vi "Outputs.vi"(8 "error in (no error)":errorcluster, 11 "State in":T1={"State"=enum."Idle", "Start Time"=timestamp(0 s since 1904-01-01), "Configuration"={"Cycle Period"=0.0, "PID 2 Parameters"={"Input Device"=enum."4-20mA", "Output Device"=enum."Default", "Setpoint"=0.0, "PID gains"={"proportional gain (Kc)"=0.0, "integral time (Ti, min)"=0.0, "derivative time (Td, min)"=100.0}, "output range"={"output low"=0.0, "output high"=1.0}}, "Manual Entry"=0.0, "Auto?"=TRUE, "4-20mA Input Settings"={"Input Channel "=0}, "4-20mA Out Settings"={"Output DAQ Task"=""}, "Input Channel Tag Name "=""}, "Current Time"=timestamp(0 s since 1904-01-01), "PID 1 Parameters"={"Setpoint"=0.0, "PID gains"={"proportional gain (Kc)"=1.0, "integral time (Ti, min)"=0.01, "derivative time (Td, min)"=0.0}}, "First Iteration"=FALSE, "Data"={"4-20mA Input"=0.0, "PID 2 Process Variable"=0.0, "PID 2 Output"=0.0, "4-20mA Output"=0.0}, "Process Name"="", "Pump On?"=enum."Off", "Input Error"=FALSE, "Output Error"=FALSE, "Log Started"=FALSE, "Current Setpoint"=0.0} {"Configuration"."PID 2 Parameters"."output range"."output low" format="%.2f"; "Configuration"."PID 2 Parameters"."output range"."output high" min=0.0 max=100.0 format="%.2f"; "Configuration"."PID 2 Parameters"."PID gains"."derivative time (Td, min)" format="%.3f"; "Configuration"."PID 2 Parameters"."PID gains"."integral time (Ti, min)" format="%.3f"; "Configuration"."PID 2 Parameters"."PID gains"."proportional gain (Kc)" format="%.3f"; "PID 1 Parameters"."PID gains"."derivative time (Td, min)" format="%.3f"; "PID 1 Parameters"."PID gains"."integral time (Ti, min)" format="%.3f"; "PID 1 Parameters"."PID gains"."proportional gain (Kc)" format="%.3f"}) -> (0 "error out":errorcluster, 3 "State out":T1={"State"=enum."Idle", "Start Time"=timestamp(0 s since 1904-01-01), "Configuration"={"Cycle Period"=0.0, "PID 2 Parameters"={"Input Device"=enum."4-20mA", "Output Device"=enum."Default", "Setpoint"=0.0, "PID gains"={"proportional gain (Kc)"=0.0, "integral time (Ti, min)"=0.0, "derivative time (Td, min)"=100.0}, "output range"={"output low"=0.0, "output high"=1.0}}, "Manual Entry"=0.0, "Auto?"=TRUE, "4-20mA Input Settings"={"Input Channel "=0}, "4-20mA Out Settings"={"Output DAQ Task"=""}, "Input Channel Tag Name "=""}, "Current Time"=timestamp(0 s since 1904-01-01), "PID 1 Parameters"={"Setpoint"=0.0, "PID gains"={"proportional gain (Kc)"=1.0, "integral time (Ti, min)"=0.01, "derivative time (Td, min)"=0.0}}, "First Iteration"=FALSE, "Data"={"4-20mA Input"=0.0, "PID 2 Process Variable"=0.0, "PID 2 Output"=0.0, "4-20mA Output"=0.0}, "Process Name"="", "Pump On?"=enum."Off", "Input Error"=FALSE, "Output Error"=FALSE, "Log Started"=FALSE, "Current Setpoint"=0.0} {"Configuration"."PID 2 Parameters"."output range"."output low" format="%.2f"; "Configuration"."PID 2 Parameters"."output range"."output high" min=0.0 max=100.0 format="%.2f"; "Configuration"."PID 2 Parameters"."PID gains"."derivative time (Td, min)" format="%.3f"; "Configuration"."PID 2 Parameters"."PID gains"."integral time (Ti, min)" format="%.3f"; "Configuration"."PID 2 Parameters"."PID gains"."proportional gain (Kc)" format="%.3f"; "PID 1 Parameters"."PID gains"."derivative time (Td, min)" format="%.3f"; "PID 1 Parameters"."PID gains"."integral time (Ti, min)" format="%.3f"; "PID 1 Parameters"."PID gains"."proportional gain (Kc)" format="%.3f"})   [LabVIEW 2018, in "4-20mA Module.lvlib" / "4-20mA Module Engine.lvlib"]
uses:
  4-20mA Module Engine.lvlib
  State Cluster.ctl
  State Enum.ctl
  Pressure Transmitter/Pressure Transmitter Device Settings.ctl
  Pressure Reg Module/Pressure Regulator Device Settings.ctl
  Measure Instrument/PID 1 Parameters Cluster.ctl
  Tag VIs/Tag FGV Operation Enum.ctl
  Shared Variables/Dynamic Shared Variables.lvlib
  Pressure Reg Module/Pressure Regulator Library.lvlib
  Flow Regulator/Pressure Reg Module/Flow Regulator Library.lvlib
  Pressure Transmitter/Pressure Transmitter Library.lvlib
panel:
  # "Instrument Settings"
  # "Instrument Settings"
  # "Instrument Settings"
  # "Instrument Settings"
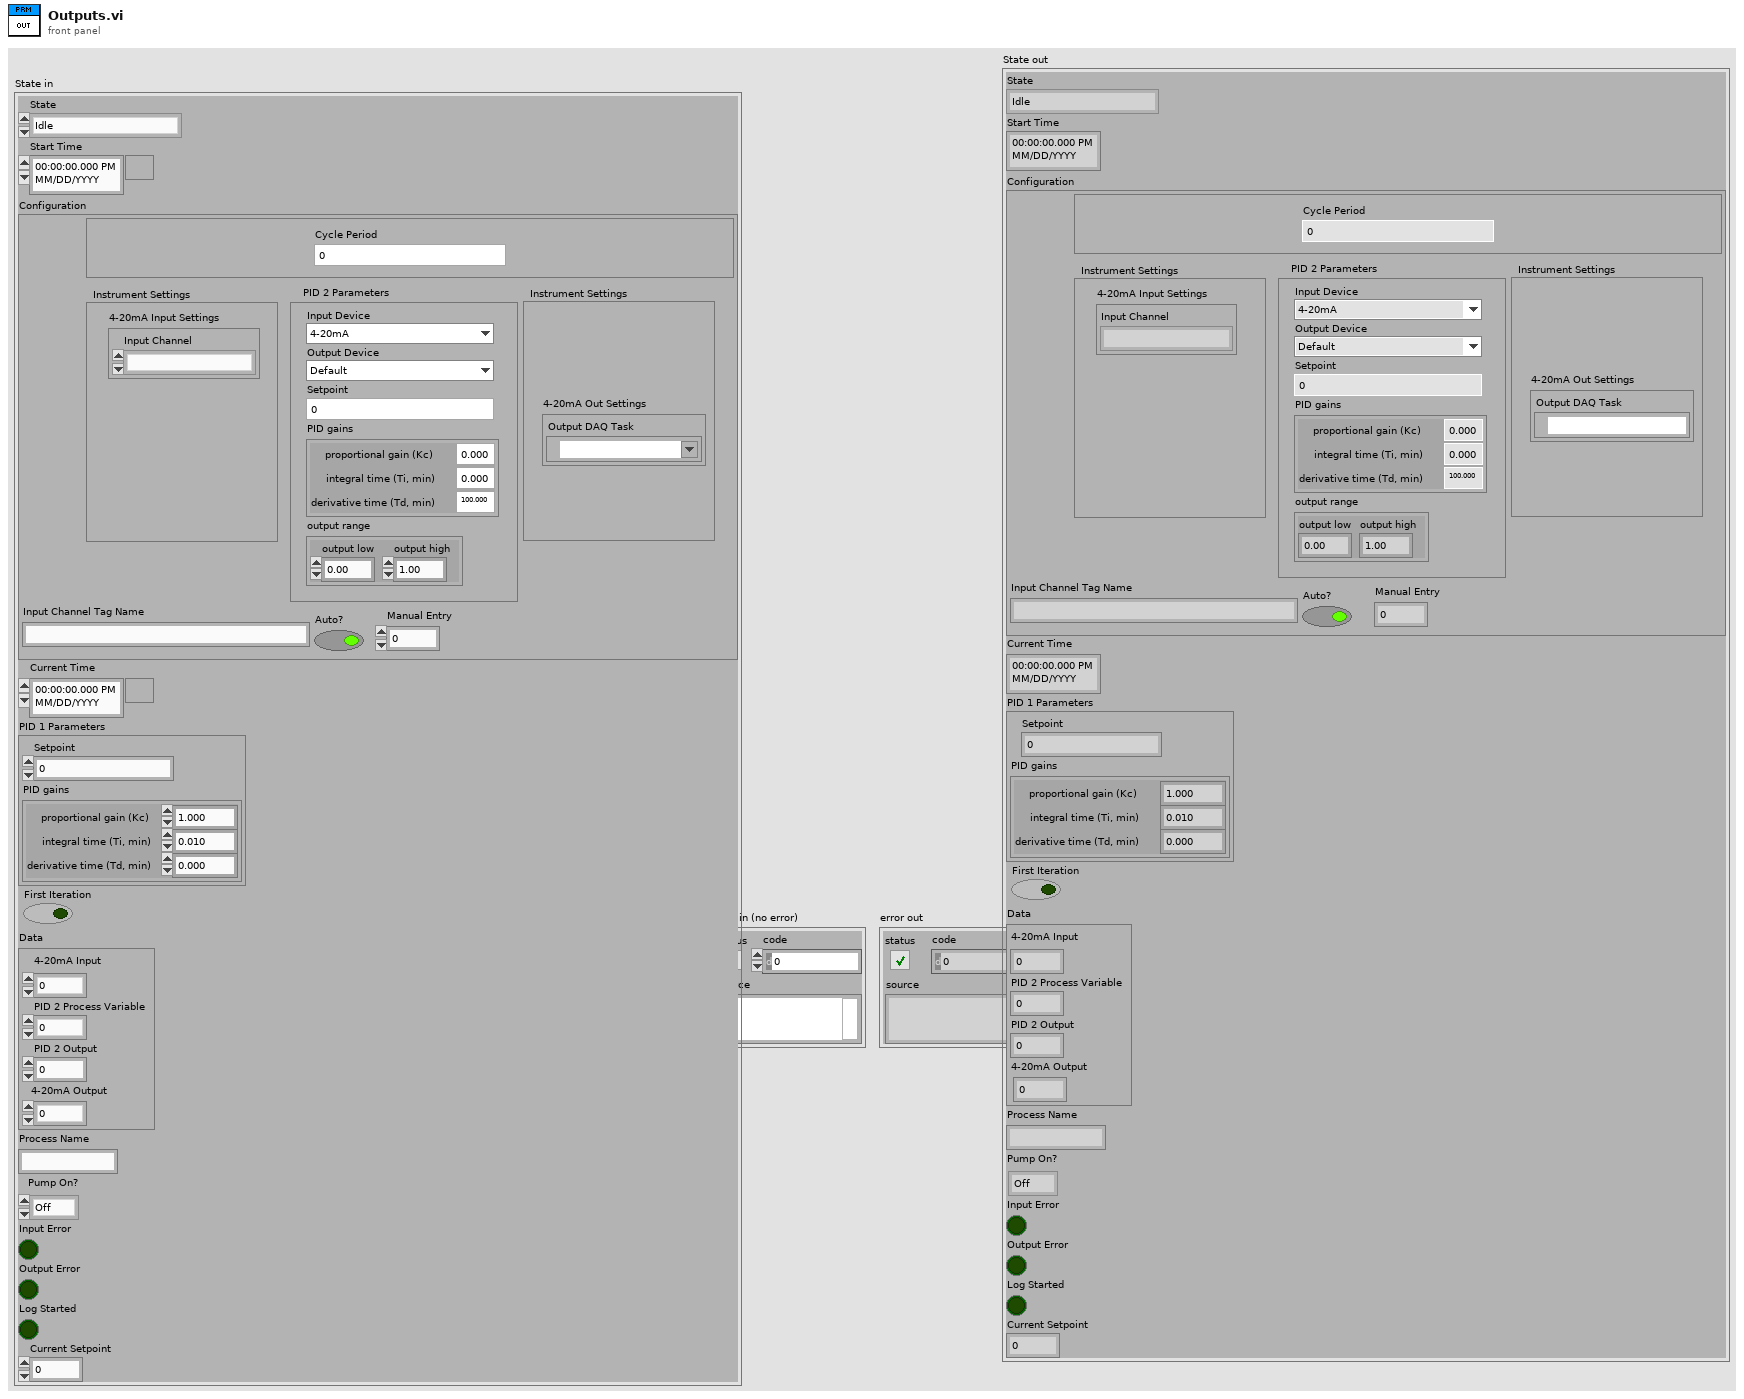
[diagram p1: front panel]
types:
  T1 = typedef "4-20mA Module.lvlib/4-20mA Module Engine.lvlib/State Cluster.ctl" = cluster{"State":T2, "Start Time":timestamp, "Configuration":cluster{"Cycle Period":dbl, "PID 2 Parameters":cluster{"Input Device":enum16{"Default", "4-20mA"}, "Output Device":enum16{"Default", "Equilibar Pressure Reg", "Flow Regulator"}, "Setpoint":dbl, "PID gains":cluster{"proportional gain (Kc)":dbl, "integral time (Ti, min)":dbl, "derivative time (Td, min)":dbl}, "output range":cluster{"output low":dbl, "output high":dbl}}, "Manual Entry":dbl, "Auto?":bool, "4-20mA Input Settings":T3, "4-20mA Out Settings":T4, "Input Channel Tag Name ":string}, "Current Time":timestamp, "PID 1 Parameters":T5, "First Iteration":bool, "Data":cluster{"4-20mA Input":dbl, "PID 2 Process Variable":dbl, "PID 2 Output":dbl, "4-20mA Output":dbl}, "Process Name":string, "Pump On?":enum16{"Off", "On", "Not Initialized"}, "Input Error":bool, "Output Error":bool, "Log Started":bool, "Current Setpoint":dbl}
  T2 = typedef "4-20mA Module.lvlib/4-20mA Module Engine.lvlib/State Enum.ctl" = enum16{"Measuring", "Idle", "Paused"}
  T3 = typedef "Pressure Transmitter Library.lvlib/Pressure Transmitter Device Settings.ctl" = cluster{"Input Channel ":u16}
  T4 = typedef "Pressure Regulator Library.lvlib/Pressure Regulator Device Settings.ctl" = cluster{"Output DAQ Task":refnum<k21>}
  T5 = typedef "PID 1 Parameters Cluster.ctl" = cluster{"Setpoint":dbl, "PID gains":cluster{"proportional gain (Kc)":dbl, "integral time (Ti, min)":dbl, "derivative time (Td, min)":dbl}}
  T6 = typedef "Tag FGV Operation Enum.ctl" = enum16{"Init", "Set Notification Queue", "Create Tag", "Commit", "Write Tag (Numeric)", "Write Tag (Boolean)", "Read All Tags", "Read One Tag", "Delete Tag Category", "Set Alarm Parameters (Numeric)", "Set Alarm Parameters (Boolean)", "Enable All Alarms", "Disable All Alarms", "Delete All Tags", "Read Alarms", "Ack Alarm", "Read Alarm Parameters (Numeric)", "Read Alarm Parameters (Boolean)"}
  T7 = enum16{"Default", "Equilibar Pressure Reg", "Flow Regulator"}
  T8 = typedef "4-20mA Module.lvlib/4-20mA Module Tag Names Cluster.ctl" = cluster{"4-20mA Input":string, "PID 2 Out Tag":string, "4-20mA Output":string, "Input Device Tag":string, "Output Device Tag":string}
  T9 = typedef "Flow Regulator Library.lvlib/Pressure Regulator Device Settings.ctl" = cluster{"Output DAQ Task":refnum<k21>}
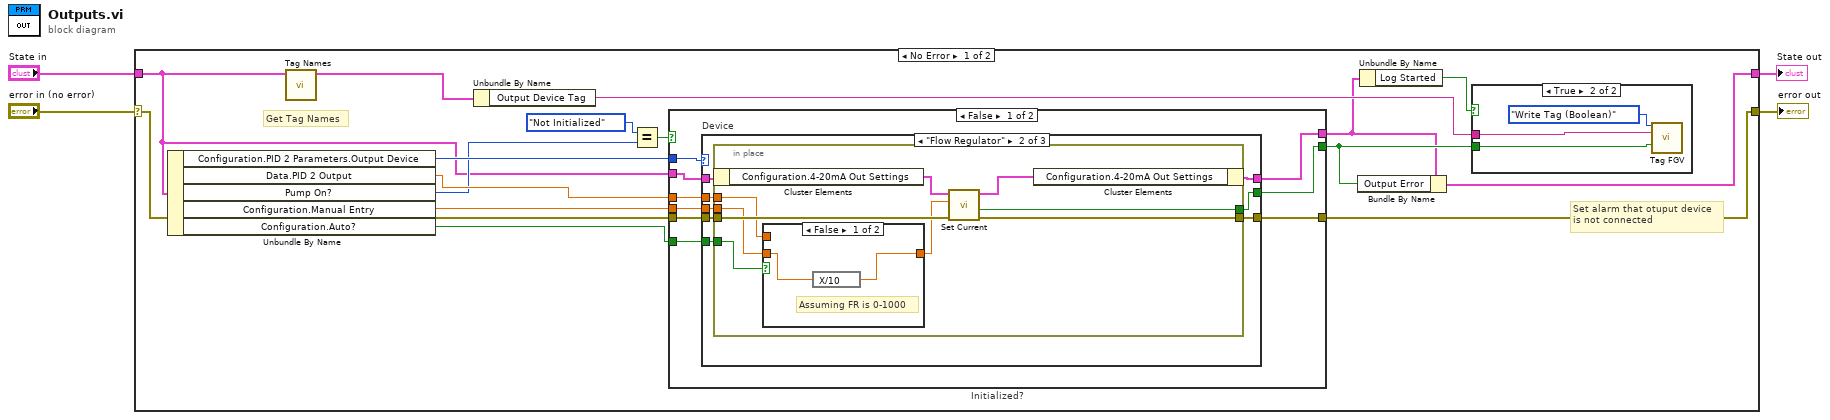
[diagram p0: block diagram]
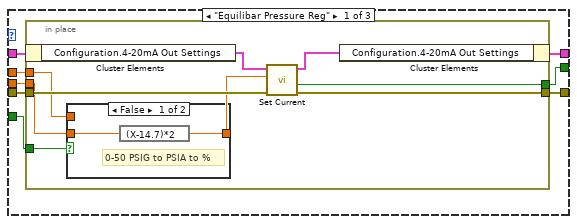
[diagram p3: hidden frame]
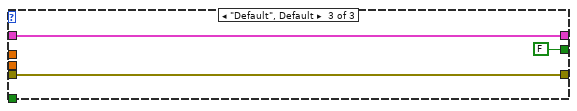
[diagram p6: hidden frame]
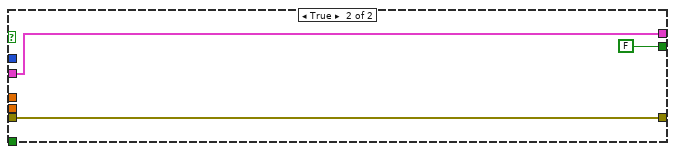
[diagram p7: hidden frame]
diagram:
  n1 = case shown="No Error" "error in (no error)" {
    selector: "error in (no error)" -> [w18 w80]
    tunnel: [w16 w80] -> w3
    tunnel: "State in" -> [w7 w79]
    tunnel: [w14 w79] -> w1
    frame No Error {
      # "Get Tag Names"
      # "Set alarm that otuput device\nis not connected"
      n2 = Unbundle By Name(w7) -> ("Configuration.PID 2 Parameters.Output Device"=w20:T7, "Data.PID 2 Output"=w19:dbl, "Pump On?"=w12:enum16{"Off", "On", "Not Initialized"}, "Configuration.Manual Entry"=w5:dbl, "Configuration.Auto?"=w6:bool)
      n3 = call "Tag Names.vi"("State in"=w7) -> ("4-20mA Module Tag Names"=w17:T8)  [unwired: 8 in, 2 out]
      n4 = Unbundle By Name(w17) -> ("Output Device Tag"=w15:string)
      n5 = Equal?(x=enum16{"Off", "On", "Not Initialized"}."Not Initialized", y=w12) -> (x = y?=w10:bool)
      n6 = case "Initialized?" shown="False" w10 {
        tunnel: w20 -> [w32 _]
        tunnel: w19 -> [w31 _]
        tunnel: w18 -> [w30 w77]
        tunnel: [w29 w77] -> w16
        tunnel: w7 -> [w28 w78]
        tunnel: [w27 w78] -> w9
        tunnel: [w26 FALSE ("Connection Error")] -> w13
        tunnel: w6 -> [w25 _]
        tunnel: w5 -> [w24 _]
        frame False {
          n7 = case "Device" shown="\"Flow Regulator\"" w32 {
            tunnel: w31 -> [w37 w56 _]
            tunnel: w30 -> [w40 w60 w74]
            tunnel: [w39 w58 w74] -> w29
            tunnel: w28 -> [w34 w54 w75]
            tunnel: [w33 w53 w75] -> w27
            tunnel: [w38 w59 FALSE ("Connection Error")] -> w26
            tunnel: w25 -> [w35 w57 _]
            tunnel: w24 -> [w36 w55 _]
            frame "Equilibar Pressure Reg" {
              n8 = in-place {
                in-place-border: w40 -> [w49]
                in-place-border: [w48] -> w39
                in-place-border: [w47] -> w38
                in-place-border: w37 -> [w46]
                in-place-border: w36 -> [w45]
                in-place-border: w35 -> [w43]
                n9 = in-place-cluster #1(w34) -> ("Configuration.4-20mA Out Settings"=w42:T4)
                n10 = case shown="False" w43 {
                  tunnel: w46 -> [_ w52]
                  tunnel: [w51 w52] -> w44
                  tunnel: w45 -> [w50 _]
                  frame False {
                    # "0-50 PSIG to PSIA to %"
                    n11 = expression code="(X-14.7)*2"(w50) -> (w51:dbl)
                  }
                  frame True {
                  }
                }
                n12 = call "Set Current.vi"("error in"=w49, "%"=w44, "4-20mA Out Settings In"=w42) -> ("error out"=w48:errorcluster, "Connection Error"=w47:bool, "4-20mA Out Settings Out"=w41:T4)  [unwired: 6 in]
                n13 = in-place-cluster #1("Configuration.4-20mA Out Settings"=w41) -> (w33:T1)
              }
            }
            frame "Flow Regulator" {
              n14 = in-place {
                in-place-border: w60 -> [w69]
                in-place-border: [w68] -> w59
                in-place-border: [w67] -> w58
                in-place-border: w57 -> [w66]
                in-place-border: w56 -> [w65]
                in-place-border: w55 -> [w63]
                n15 = in-place-cluster #2(w54) -> ("Configuration.4-20mA Out Settings"=w62:T4)
                n16 = case shown="False" w66 {
                  tunnel: w65 -> [_ w72]
                  tunnel: [w71 w72] -> w64
                  tunnel: w63 -> [w70 _]
                  frame False {
                    # "Assuming FR is 0-1000"
                    n17 = expression code="X/10"(w70) -> (w71:dbl)
                  }
                  frame True {
                  }
                }
                n18 = call "Set Current.vi"("error in"=w69, "%"=w64, "4-20mA Out Settings In"=w62) -> ("error out"=w67:errorcluster, "Connection Error"=w68:bool, "4-20mA Out Settings Out"=w61:T9)  [unwired: 6 in]
                n19 = in-place-cluster #2("Configuration.4-20mA Out Settings"=w61) -> (w53:T1)
              }
            }
            frame "Default", Default {
            }
          }
        }
        frame True {
        }
      }
      n20 = Bundle By Name(cluster=w9, "Output Error"=w13) -> (w14:T1)
      n21 = Unbundle By Name(w9) -> ("Log Started"=w8:bool)
      n22 = case shown="True" w8 {
        tunnel: w15 -> [_ w23]
        tunnel: w13 -> [_ w21]
        frame False {
        }
        frame True {
          n23 = call "Tag FGV.vi"("Operation"=Tag_FGV_Operation_Enum."Write Tag (Boolean)", "Tag Name"=w23, "Data"=w21) -> ()  [unwired: 5 in, 8 out]
        }
      }
    }
    frame Error {
    }
  }
  "error out" <- w3
  "State out" <- w1
